vi "285_SetVelRes_velres.vi"(8 "error in (no error)":errorcluster caption="错误输入（无错误）", 10 "速度":dbl, 11 "精度":u16(ring)=10 items=["Low (10microsteps/step)", "High (50microsteps/step)"]) -> (0 "error out":errorcluster caption="错误输出")   [LabVIEW 2016]
uses:
  <vilib>/Instr/_visa.llb/VISA Configure Serial Port (Instr).vi
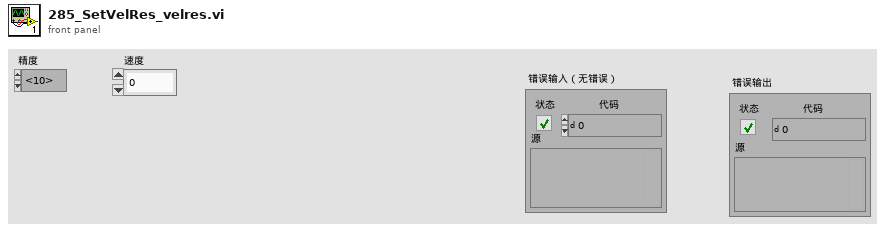
[diagram p1: front panel]
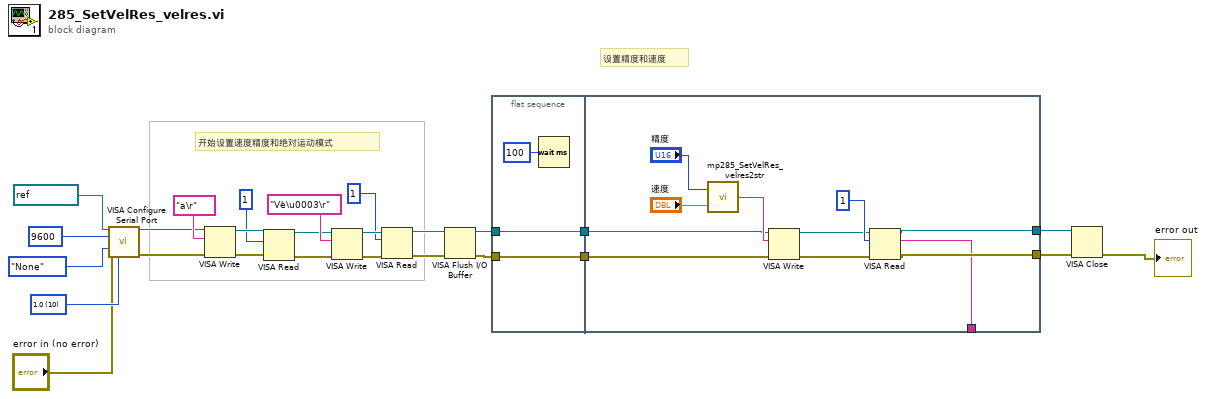
[diagram p0: block diagram]
diagram:
  w5 = u16 10 items=["1.0"=10, "1.5"=15, "2.0"=20] ("停止位 (10: 1位)")
  # "开始设置速度精度和绝对运动模式"
  # "设置精度和速度"
  n1 = call-poly "VISA Configure Serial Port"("VISA resource name"=refnum<visa-resource-name> "COM4" ("VISA资源名称"), "baud rate (9600)"=u32 9600 ("波特率(9600)"), "parity (0:none)"=enum16{"None", "Odd", "Even", "Mark", "Space"}."None" ("校验（无）"), "error in (no error)"="error in (no error)", "stop bits (10: 1 bit)"=w5) -> ("VISA resource name out"=w12:refnum<visa-resource-name>, "error out"=w11:errorcluster)  [unwired: 9 in]
  n2 = VISA Write ("VISA写入")(VISA resource name=w12, write buffer="a\r" ("写入缓冲区"), error in (no error)=w11) -> (VISA resource name out=w19:refnum<visa-resource-name>, error out=w20:errorcluster)  [unwired: 1 out]
  n3 = VISA Read(VISA resource name=w19, byte count=u32 1 ("字节总数"), error in (no error)=w20) -> (VISA resource name out=w18:refnum<visa-resource-name>, error out=w17:errorcluster)  [unwired: 2 out]
  n4 = VISA Write ("VISA写入")(VISA resource name=w18, write buffer="Vè\u0003\r" ("写入缓冲区"), error in (no error)=w17) -> (VISA resource name out=w14:refnum<visa-resource-name>, error out=w15:errorcluster)  [unwired: 1 out]
  n5 = VISA Read(VISA resource name=w14, byte count=u32 1 ("字节总数"), error in (no error)=w15) -> (VISA resource name out=w9:refnum<visa-resource-name>, error out=w10:errorcluster)  [unwired: 2 out]
  n6 = VISA Flush I/O Buffer(VISA resource name=w9, error in (no error)=w10) -> (VISA resource name out=w4:refnum<visa-resource-name>, error out=w3:errorcluster)  [unwired: 1 in]
  n7 = flat-sequence {
    tunnel: w3 -> [w28]
    tunnel: w4 -> [w29]
    tunnel: [w29] -> w26
    tunnel: [w28] -> w25
    tunnel: [w32] -> w24
    tunnel: [w31] -> w23
    tunnel: [w30] -> _
    tunnel: w26 -> [w36]
    tunnel: w25 -> [w35]
    frame #0 {
      n8 = Wait (ms)(milliseconds to wait=u32 100 ("等待时间（毫秒）")) -> ()  [unwired: 1 out]
    }
    frame #1 {
      n9 = call "mp285_SetVelRes_velres2str.vi"("速度"="速度", "精度"="精度") -> ("发送至串口的字符串"=w37:string)
      n10 = VISA Write ("VISA写入")(VISA resource name=w36, write buffer=w37, error in (no error)=w35) -> (VISA resource name out=w39:refnum<visa-resource-name>, error out=w38:errorcluster)  [unwired: 1 out]
      n11 = VISA Read(VISA resource name=w39, byte count=u32 1 ("字节总数"), error in (no error)=w38) -> (VISA resource name out=w32:refnum<visa-resource-name>, read buffer=w30:string, error out=w31:errorcluster)  [unwired: 1 out]
    }
  }
  n12 = VISA Close(VISA resource name=w24, error in (no error)=w23) -> (error out=→"error out":errorcluster)
